vi "SAOMM-HexapodOffsets.vi"() -> ()   [LabVIEW 2011]
panel:
  out "Offset":T1
  out "Position":T2
  in  "-X 5":bool
  in  "+X 5":bool
  in  "-X 4":bool
  in  "+X 4":bool
  in  "-X 3":bool
  in  "+X 3":bool
  in  "-Y":bool
  in  "+Y":bool
  in  "-X":bool
  in  "+X":bool
  in  "Quit":bool
  in  "Apply":bool
  out "Off V":dbl caption="Pos" format="%.6f"
  out "Off U":dbl caption="Pos" format="%.6f"
  out "Off Z":dbl caption="Pos" format="%.6f"
  out "Off Y":dbl caption="Pos" format="%.6f"
  out "Off X":dbl caption="Pos" format="%.6f"
  out "Pos V":dbl caption="Pos" format="%.6f"
  out "Pos U":dbl caption="Pos" format="%.6f"
  out "Pos Z":dbl caption="Pos" format="%.6f"
  out "Pos Y":dbl caption="Pos" format="%.6f"
  out "Pos X":dbl caption="Pos" format="%.6f"
  # "/"
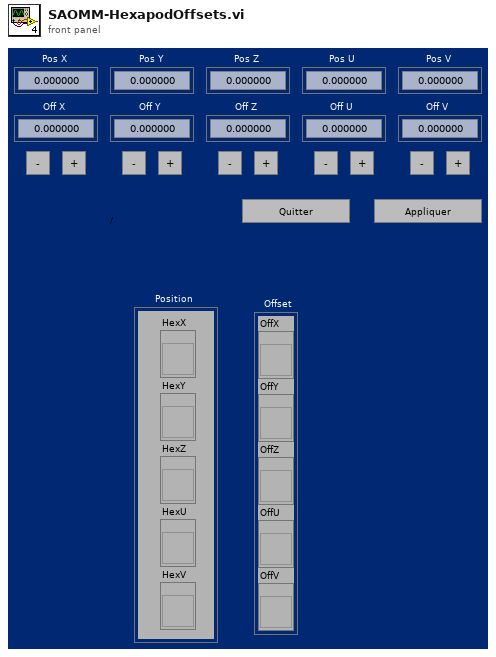
[diagram p1: front panel]
types:
  T1 = cluster{"OffX":refnum<vi>, "OffY":refnum<vi>, "OffZ":refnum<vi>, "OffU":refnum<vi>, "OffV":refnum<vi>}
  T2 = cluster{"HexX":refnum<vi>, "HexY":refnum<vi>, "HexZ":refnum<vi>, "HexU":refnum<vi>, "HexV":refnum<vi>}
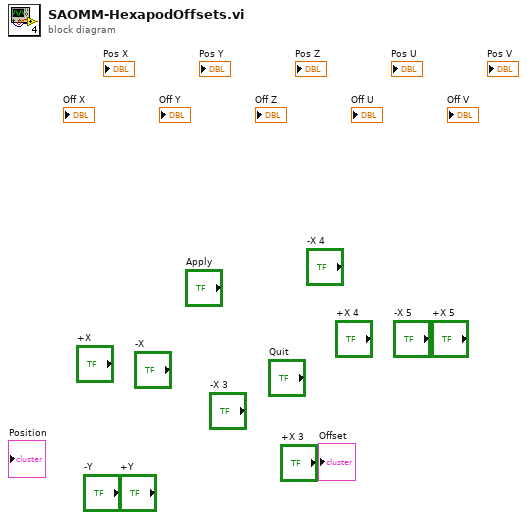
[diagram p0: block diagram]
diagram:
